vi "FTW-File-GetShellIcon.vi"(0 "Filepath":path, 11 "error in":errorcluster) -> (4 "Icon":picture, 15 "error out":errorcluster)   [LabVIEW 2014]
uses:
  core/ui/image/FTW-Image-AppendToPicture.vi
panel:
  # "Inputs"
  # "Outputs"
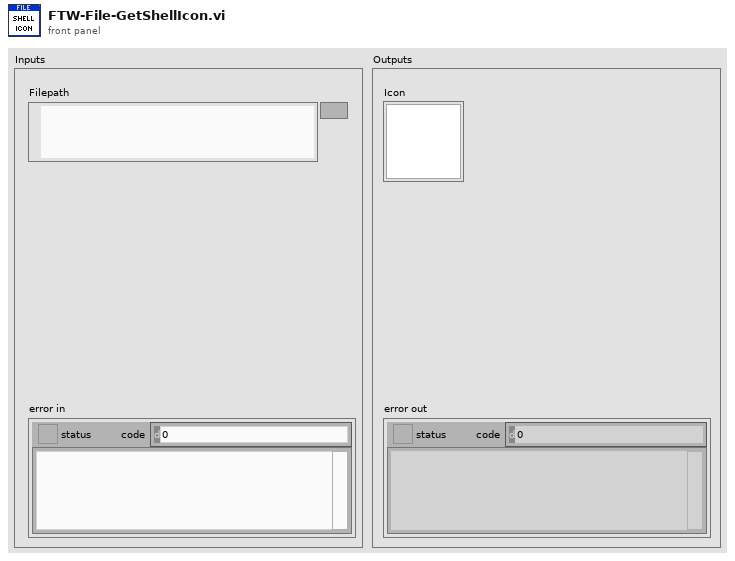
[diagram p1: front panel]
types:
  T1 = typedef "imagedata.ctl" = cluster{"image type":i32, "image depth":i32, "image":u8[], "mask":u8[], "colors":u32[], "Rectangle":cluster{"left":i16, "top":i16, "right":i16, "bottom":i16}}
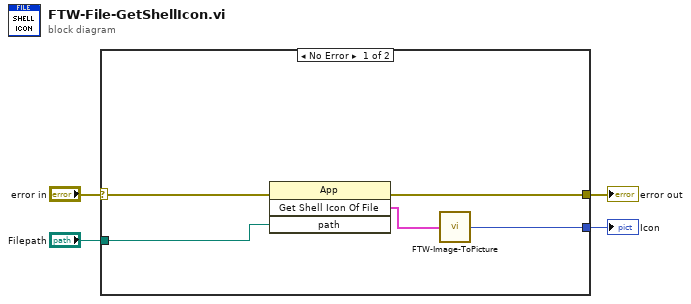
[diagram p0: block diagram]
diagram:
  n1 = case shown="No Error" "error in" {
    selector: "error in" -> [w9 w10]
    tunnel: "Filepath" -> [w7 _]
    tunnel: [w8 w10] -> w2
    tunnel: [w5 _] -> w1
    frame No Error {
      n2 = invoke class="App" method="Get Shell Icon Of File"(error in=w9, "path"=w7) -> (error out=w8:errorcluster, "GetShellIconOfFile"=w6:T1)  [unwired: 2 in, 2 out]
      n3 = call "FTW-Image-ToPicture.vi"("Image"=w6) -> ("Picture"=w5:picture)
    }
    frame Error {
    }
  }
  "error out" <- w2
  "Icon" <- w1
